vi "AIT 1553 - Create BC Sysdef Tree Messages.vi"(7 "Called From SysDef API (F)":bool, 8 "error in":errorcluster, 9 "BC Messages":T1[](array[typedef]), 10 "Section Ptr":T3 format="%.0x") -> (0 "error out":errorcluster)   [LabVIEW 2013]
uses:
  <vilib>/NI Veristand/Custom Device API/Custom Device Item Ref.ctl
  Controls/1553_BC_Message.ctl
  Controls/664 -Param.ctl
  <vilib>/NI Veristand/Custom Device API/Custom Device Channel Type.ctl
  <vilib>/NI Veristand/Custom Device API/Custom Device Channel.ctl
  Controls and Global/Global.vi
  <vilib>/NI Veristand/Custom Device API/Custom Device API.lvlib
  AIT 664 Custom Device.lvlib
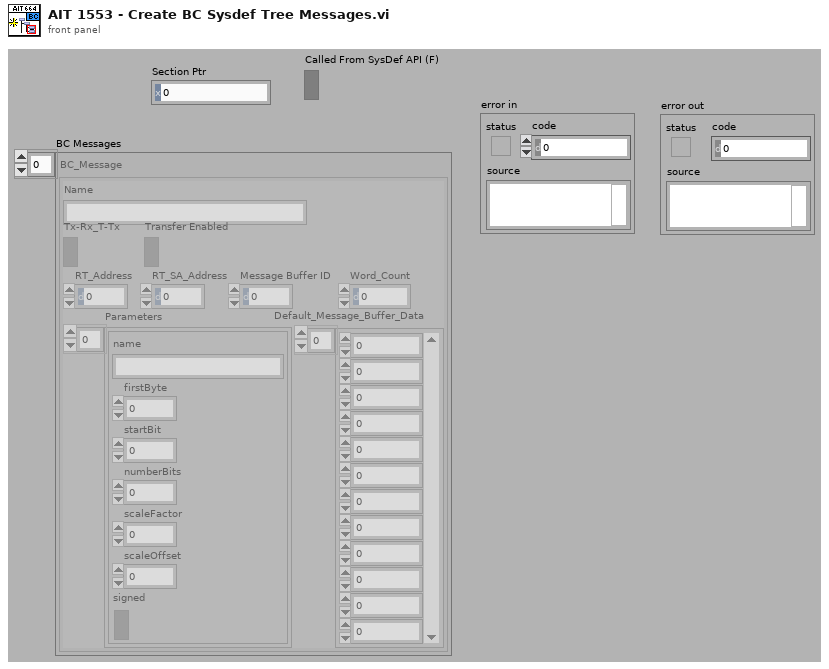
[diagram p1: front panel]
types:
  T1 = typedef "AIT 664 Custom Device.lvlib/1553_BC_Message.ctl" = cluster{"Name":string, "Tx-Rx_T-Tx":bool, "RT_Address":u8, "RT_SA_Address":u8, "Parameters":T2[], "Transfer Enabled":bool, "Message Buffer ID":u16, "Default_Message_Buffer_Data":u16[], "Word_Count":u8}
  T2 = typedef "AIT 664 Custom Device.lvlib/664 -Param.ctl" = cluster{"name":string, "firstByte":i32, "startBit":i32, "numberBits":i32, "scaleFactor":dbl, "scaleOffset":dbl, "signed":bool}
  T3 = typedef "Custom Device API.lvlib/Custom Device Item Ref.ctl" = u64
  T4 = typedef "Custom Device API.lvlib/Custom Device Channel.ctl" = cluster{"Type":T5, "Units":string, "Default Value":dbl, "Faultable":bool, "Scalable":bool}
  T5 = typedef "Custom Device API.lvlib/Custom Device Channel Type.ctl" = enum16{"Input", "Output"}
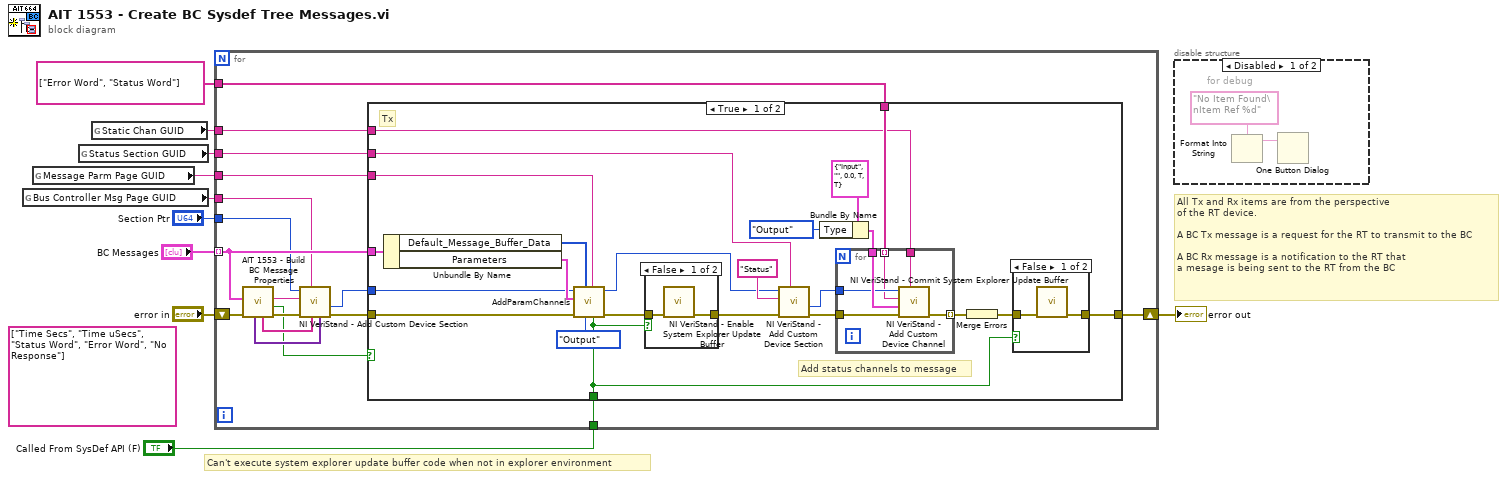
[diagram p0: block diagram]
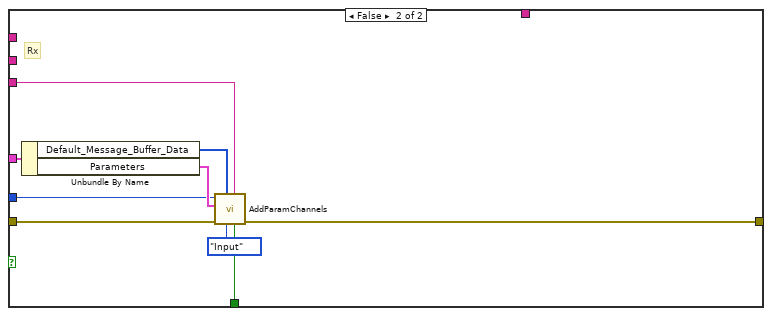
[diagram p5: hidden frame]
diagram:
  (unwired) string[] ["Time Secs", "Time uSecs", "Status Word", "Error Word", "No Response"]
  # "Can't execute system explorer update buffer code when not in explorer environment"
  # "All Tx and Rx items are from the perspective \nof the RT device.\n\nA BC Tx message is a request for the RT to transmit to the BC\n\nA BC Rx message is a notification to the RT that\na mesage is being sent to the RT from the BC"
  n1 = global read "Global.vi" "Bus Controller Msg Page GUID"() -> (w7:string)
  n2 = global read "Global.vi" "Message Parm Page GUID"() -> (w4:string)
  n3 = global read "Global.vi" "Status Section GUID"() -> (w2:string)
  n4 = global read "Global.vi" "Static Chan GUID"() -> (w6:string)
  n5 = for {
    shift-right: [w12] -> w10
    shift-left: "error in" -> [w23]
    tunnel: "Section Ptr" -> [w20]
    tunnel: "BC Messages" -> [w22] mode=indexing
    tunnel: w7 -> [w21]
    tunnel: w6 -> [w13]
    tunnel: w4 -> [w19]
    tunnel: string[] ["Error Word", "Status Word"] -> [w14]
    tunnel: w2 -> [w15]
    tunnel: "Called From SysDef API (F)" -> [w11]
    n6 = call "AIT 1553 - Build BC Message Properties.vi"("error in (no error)"=w23, "BC_Message"=w22) -> ("error out"=w25:errorcluster, "Tx-Rx  (T=Tx)"=w16:bool, "name"=w24:string, "Prop Names"=w26:string[], "Prop Values"=w27:variant[])  [unwired: 5 in]
    n7 = call <vilib>:"NI VeriStand - Add Custom Device Section.vi"("Property Values"=w27, "Property names"=w26, "GUID (Default Section)"=w21, "error in (no error)"=w25, "Section Name"=w24, "Parent Ref in"=w20) -> ("error out"=w18:errorcluster, "Section Ptr"=w17:T3)  [unwired: 2 in, 2 out]
    n8 = case shown="True" w16 {
      tunnel: w18 -> [w49 w70]
      tunnel: w17 -> [w48 w69]
      tunnel: [w33 w66] -> w12
      tunnel: w22 -> [w46 w67]
      tunnel: w19 -> [w44 w64]
      tunnel: w15 -> [w32 _]
      tunnel: w14 -> [w31 _]
      tunnel: w13 -> [w30 _]
      tunnel: w11 -> [w28 w63]
      frame True {
        # "Add status channels to message"
        # "Tx"
        n9 = Unbundle By Name(w46) -> ("Default_Message_Buffer_Data"=w45:u16[], "Parameters"=w50:T2[])
        n10 = call "AddParamChannels.vi"("Called From SysDef API (F)"=w28, "Parm Page GUID"=w44, "Type"=Custom_Device_Channel_Type."Output", "Default Message Data"=w45, "error in"=w49, "Parameters to add"=w50, "Node Ref In"=w48) -> ("error out"=w34:errorcluster, "Node Ref Out"=w29:T3)  [unwired: 3 in]
        n11 = case shown="False" w28 {
          tunnel: [w55 w56] -> w42
          tunnel: w34 -> [w54 w56]
          frame False {
            n12 = call <vilib>:"NI VeriStand - Enable System Explorer Update Buffer.vi"("error in (no error)"=w54) -> ("error out"=w55:errorcluster)  [unwired: 10 in]
          }
          frame True {
          }
        }
        n13 = call <vilib>:"NI VeriStand - Add Custom Device Section.vi"("GUID (Default Section)"=w32, "error in (no error)"=w42, "Section Name"="Status", "Parent Ref in"=w29) -> ("error out"=w39:errorcluster, "Section Ptr"=w40:T3)  [unwired: 4 in, 2 out]
        n14 = Bundle By Name(cluster=T4 {"Type"=enum."Input", "Units"="", "Default Value"=0.0, "Faultable"=TRUE, "Scalable"=TRUE} ("Channel"), "Type"=Custom_Device_Channel_Type."Output") -> (w38:T4)
        n15 = for {
          tunnel: [w62] -> w35 mode=indexing
          tunnel: w38 -> [w61]
          tunnel: w30 -> [w60]
          tunnel: w39 -> [w59]
          tunnel: w40 -> [w58]
          tunnel: w31 -> [w57] mode=indexing
          n16 = call <vilib>:"NI VeriStand - Add Custom Device Channel.vi"("GUID (Default Channel)"=w60, "error in (no error)"=w59, "Channel"=w61, "Channel Name"=w57, "Parent Ref in"=w58) -> ("error out"=w62:errorcluster)  [unwired: 3 in, 3 out]
        }
        n17 = Merge Errors(w35) -> (w43:errorcluster)
        n18 = case shown="False" w28 {
          tunnel: w43 -> [w52 w53]
          tunnel: [w51 w53] -> w33
          frame False {
            n19 = call <vilib>:"NI VeriStand - Commit System Explorer Update Buffer.vi"("error in (no error)"=w52) -> ("error out"=w51:errorcluster)  [unwired: 10 in]
          }
          frame True {
          }
        }
      }
      frame False {
        # "Rx"
        n20 = Unbundle By Name(w67) -> ("Default_Message_Buffer_Data"=w65:u16[], "Parameters"=w71:T2[])
        n21 = call "AddParamChannels.vi"("Called From SysDef API (F)"=w63, "Parm Page GUID"=w64, "Type"=Custom_Device_Channel_Type."Input", "Default Message Data"=w65, "error in"=w70, "Parameters to add"=w71, "Node Ref In"=w69) -> ("error out"=w66:errorcluster)  [unwired: 3 in, 1 out]
      }
    }
  }
  "error out" <- w10
  n22 = disable-structure shown="Disabled" {
    frame Disabled {
      # "for debug"
      n23 = Format Into String(format string="No Item Found\nItem Ref %d" ("message")) -> (resulting string=w74:string, w72:T3)  [unwired: 2 in, 1 out]
      n24 = One Button Dialog(message=w74) -> (true=w75:bool)  [unwired: 1 in]
    }
    frame Enabled {
    }
  }
